vi "Station Wise.vi"(8 "error in (no error)":errorcluster, 11 "index":i32) -> (0 "error out":errorcluster, 2 "M":bool, 3 "S":bool)   [LabVIEW 2017]
uses:
  <vilib>/addons/database/Connection.llb/DB Tools Open Connec (Path).vi
  Globle/Current date.vi
  <vilib>/addons/database/NI_Database_API.lvlib
panel:
  in  "Cancel Button":bool
  out "G Ack 2":bool
  out "GL 2":bool
  out "Table 2":string[][](array[string])
  out "Table":string[][](array[string])
  out "Duration P":dbl format="%<%M:%S>t"
  out "Duration Q":dbl format="%<%M:%S>t"
  out "Duration M":dbl format="%<%M:%S>t"
  out "Duration L":dbl format="%<%M:%S>t"
  out "Duration GL":dbl format="%<%M:%S>t"
  out "COUNT P":i32
  out "COUNT  Q":i32
  out "COUNT  M":i32
  out "COUNT  Mat":i32
  out "P Ack":bool
  out "Q Ack":bool
  out "M Ack":bool
  out "L Ack":bool
  out "G Ack":bool
  out "SS":bool
  out "Q":bool
  out "M":bool
  out "COUNT Safety":i32
  out "P Duration Min":dbl format="%<%M:%S>t"
  out "Q Duration Min":dbl format="%<%M:%S>t"
  out "M Duration Min":dbl format="%<%M:%S>t"
  out "L Duration Min":dbl format="%<%M:%S>t"
  out "GL Duration min":dbl format="%<%M:%S>t"
  out "P Counter":i32
  out "Q Counter":i32
  out "M Counter":i32
  out "Mat Counter":i32
  out "Safety Counter":i32
  # "Station Wise Live Breakdown Status"
  # "Safety"
  # "Material"
  # "Maintenance"
  # "Quality"
  # "Startup/Setup"
  # "Stakeholder"
  # "Count"
  # "Duration"
  # "Station"
  # "Breakdown Name"
  # "Safety"
  # "Min"
  # "Breakdown"
  # "Material"
  # "Min"
  # "Acknowledgement"
  # "Maintenance"
  # "Min"
  # "Total Count"
  # "Quality"
  # "Min"
  # "Total Duration (Min)"
  # "Startup/Setup"
  # "Min"
  # "Designed And Developed By - Infinity Automation Systems Pvt. Ltd."
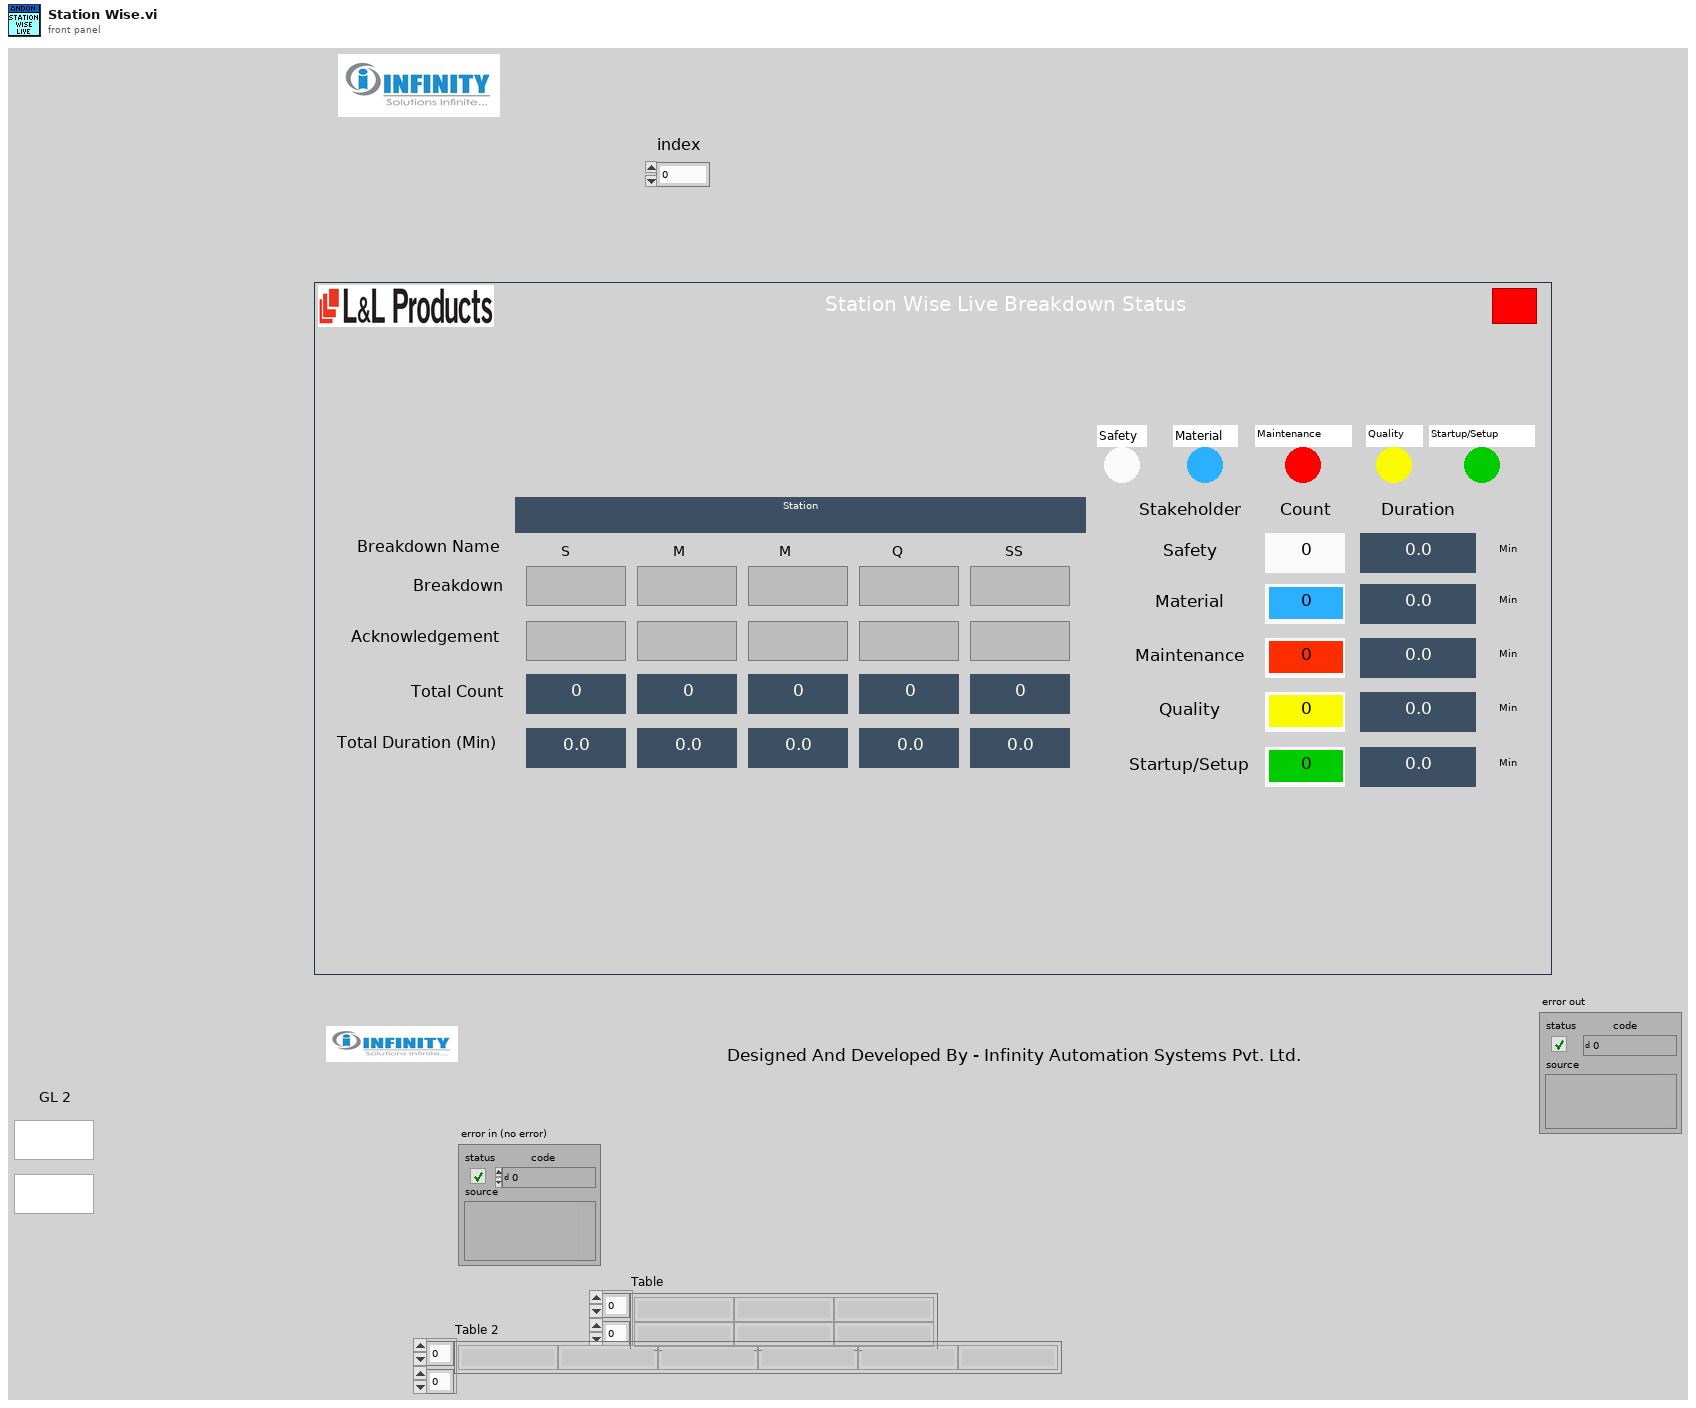
[diagram p1: front panel]
types:
  T1 = typedef "NI_Database_API.lvlib/Conn ObjectReference.ctl" = refnum<k1>
  T2 = enum32{"invalid app kind", "Development System", "Run Time System", "Student Edition", "Embedded LabVIEW", "Evaluation", "Custom"}
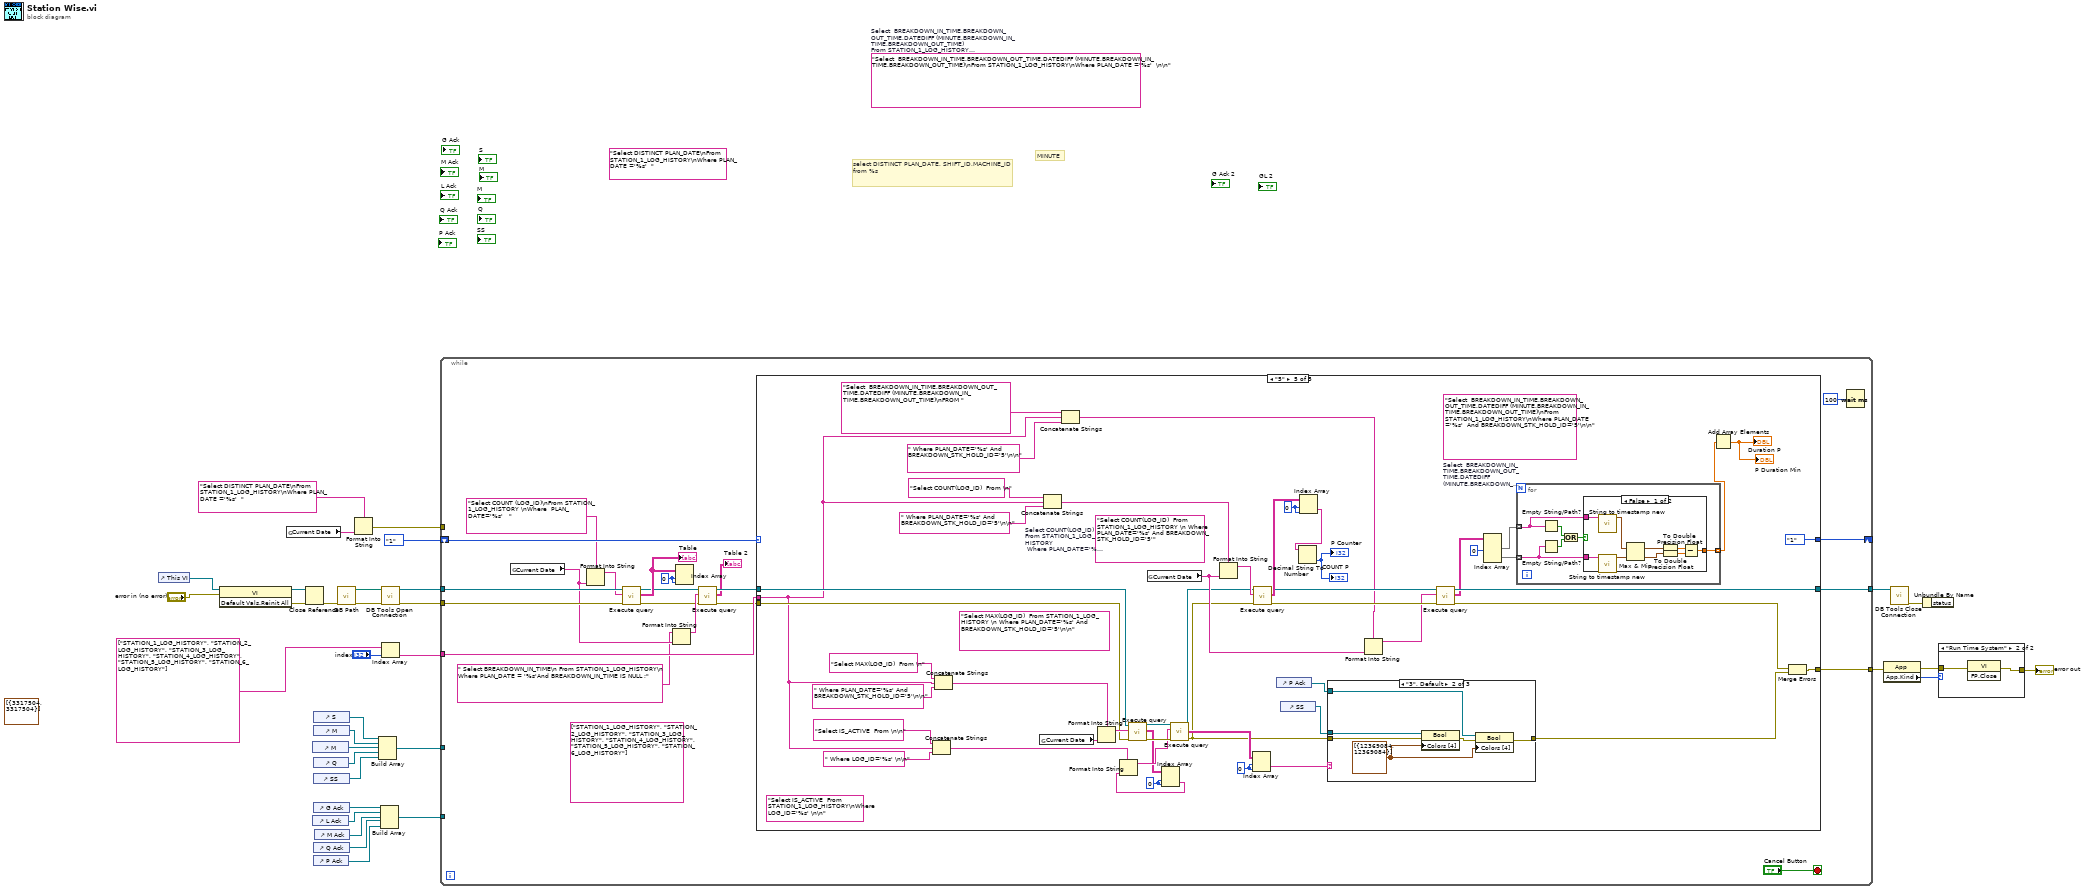
[diagram p0: block diagram]
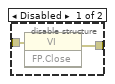
[diagram p3: hidden frame]
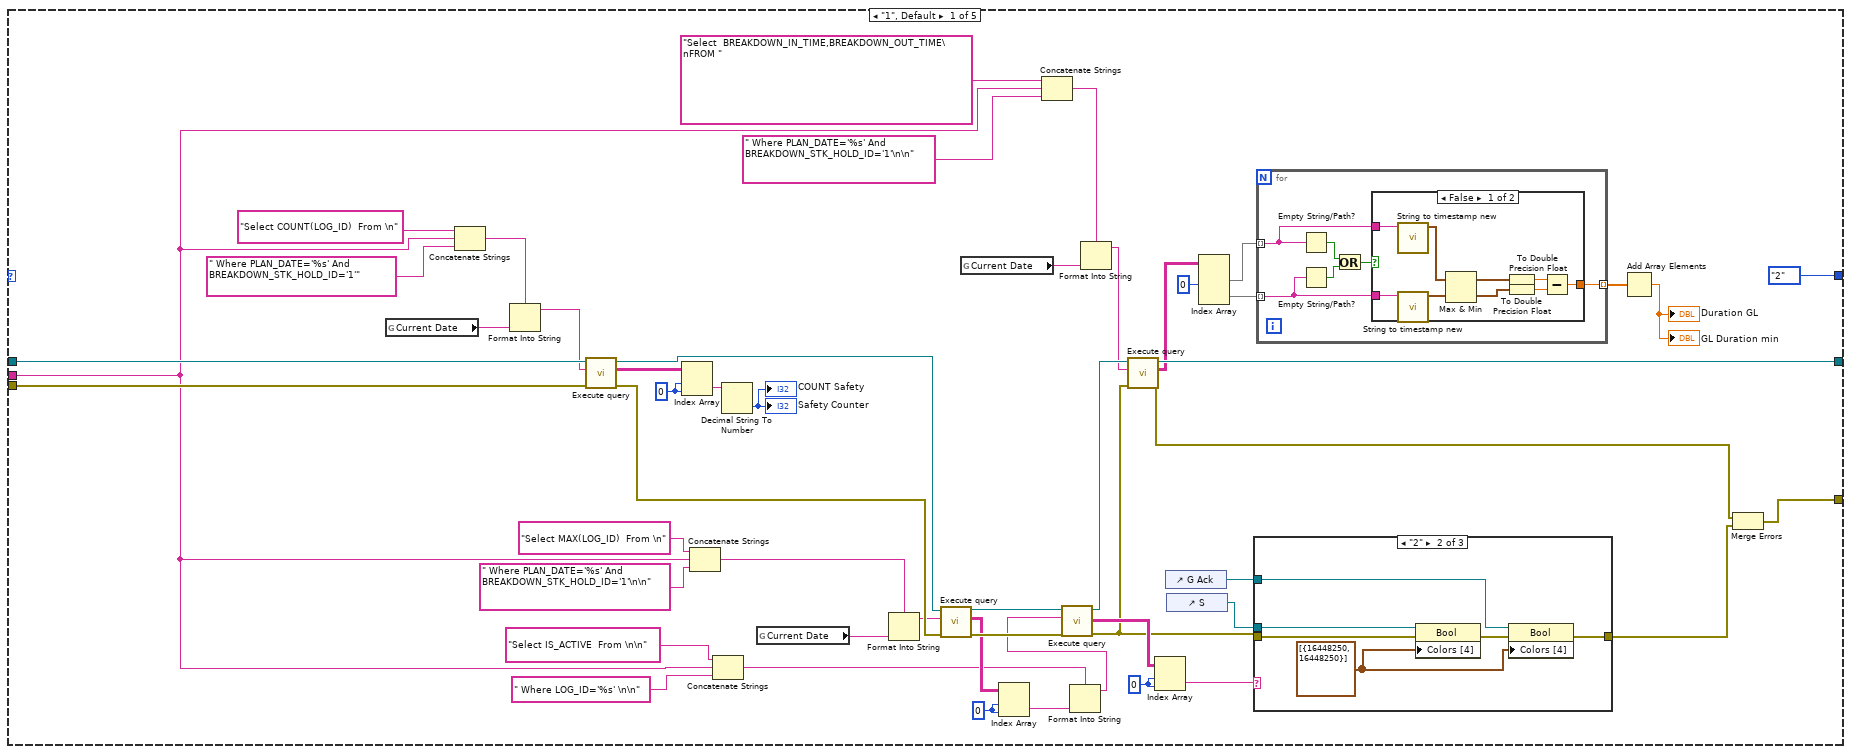
[diagram p4: hidden frame]
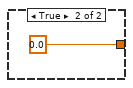
[diagram p5: hidden frame]
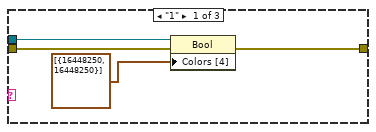
[diagram p6: hidden frame]
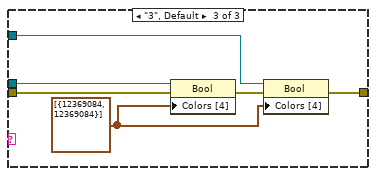
[diagram p7: hidden frame]
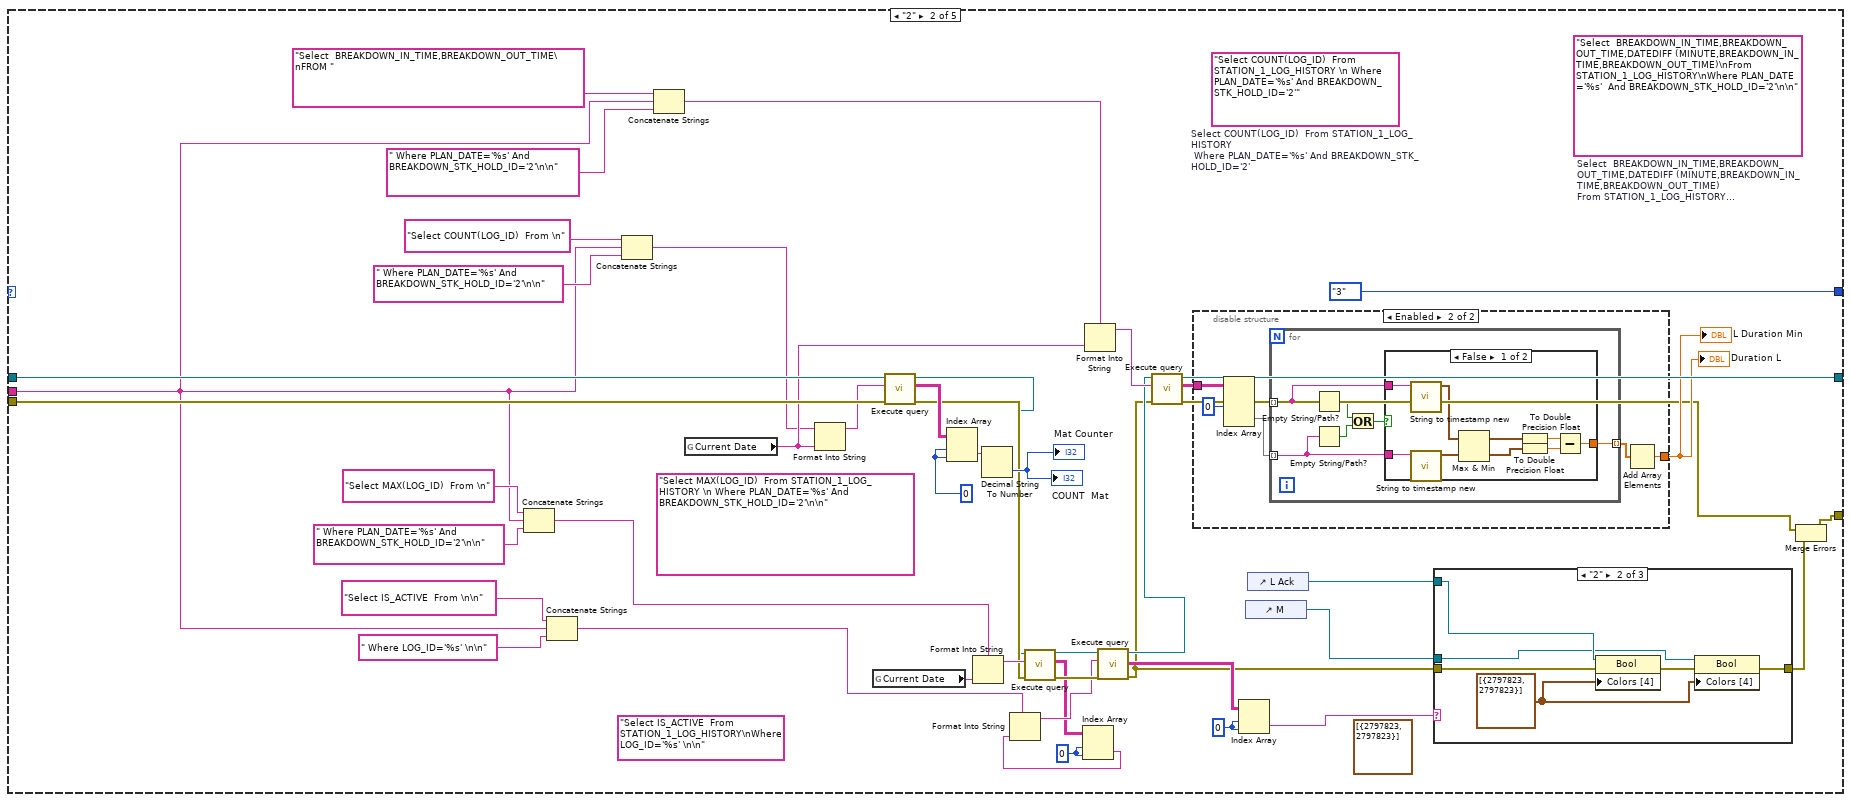
[diagram p8: hidden frame]
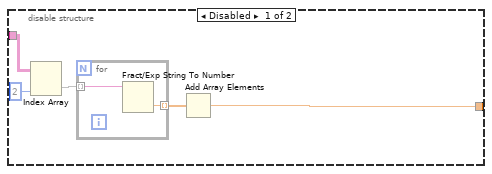
[diagram p9: hidden frame]
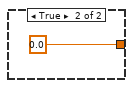
[diagram p10: hidden frame]
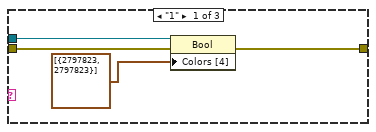
[diagram p11: hidden frame]
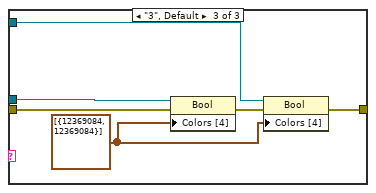
[diagram p12: hidden frame]
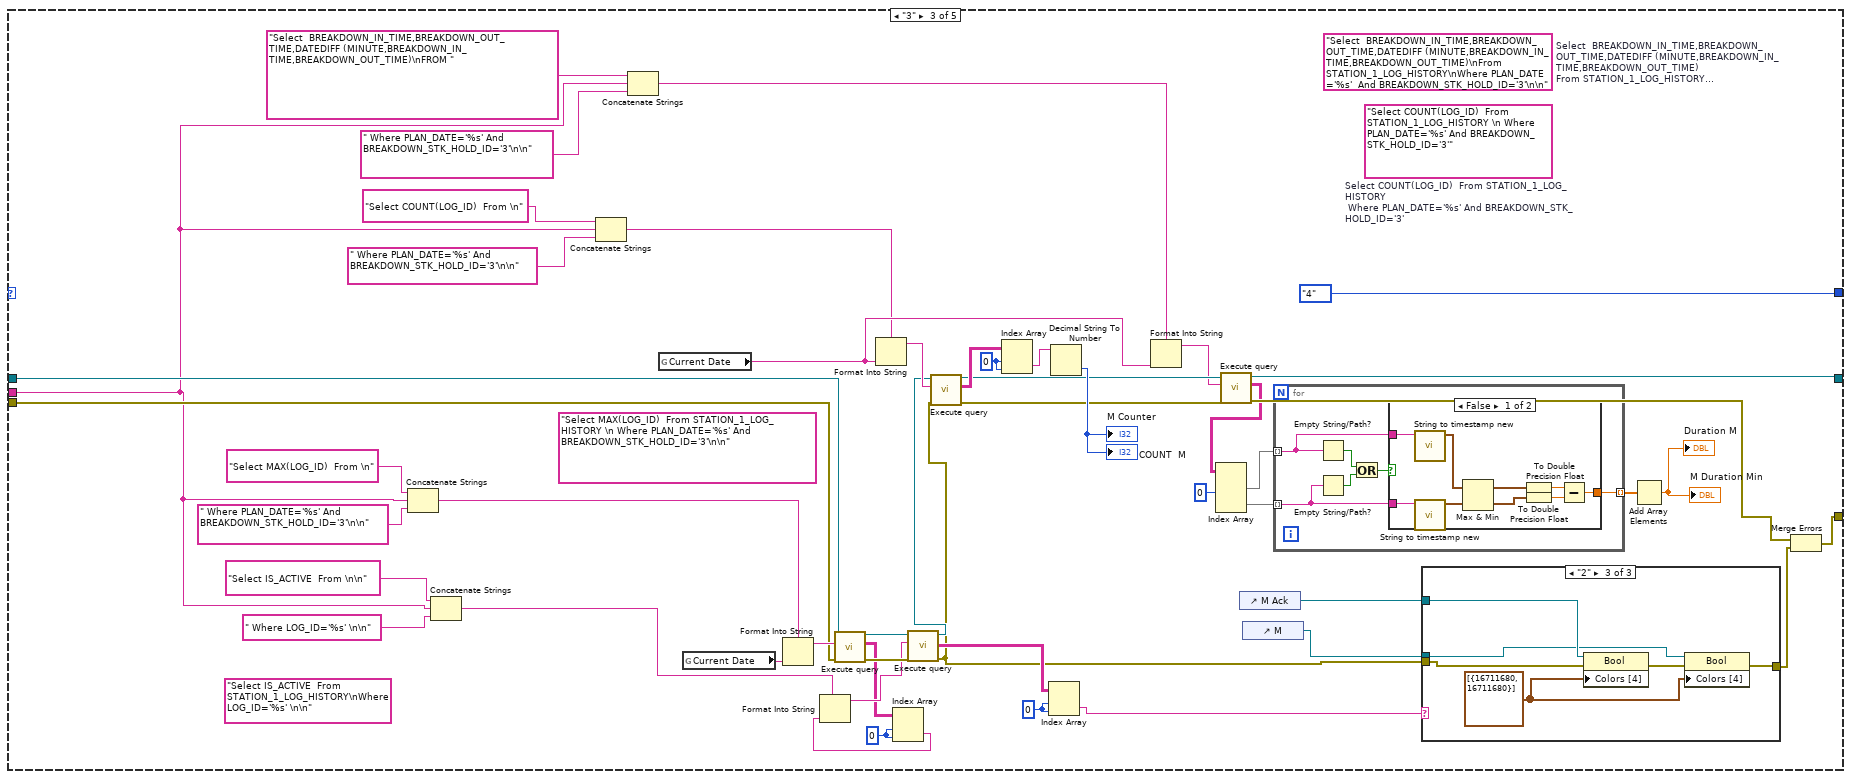
[diagram p13: hidden frame]
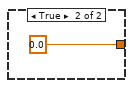
[diagram p14: hidden frame]
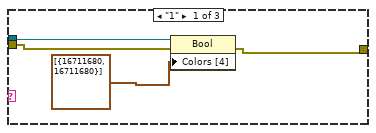
[diagram p15: hidden frame]
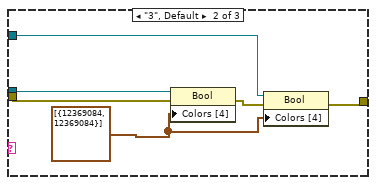
[diagram p16: hidden frame]
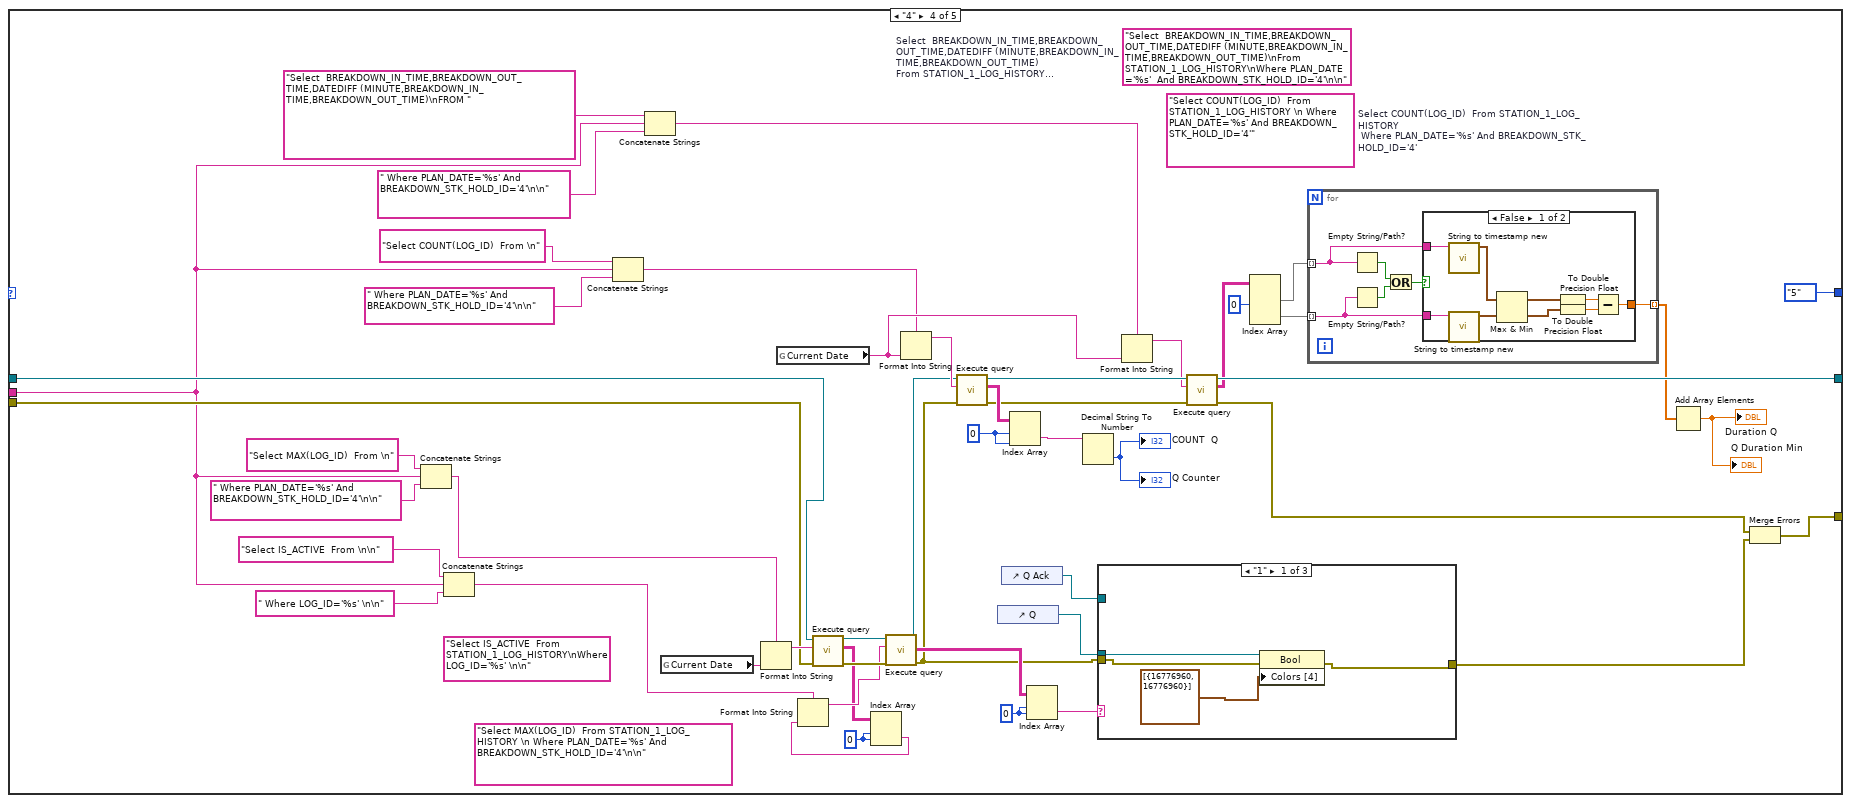
[diagram p17: hidden frame]
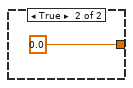
[diagram p18: hidden frame]
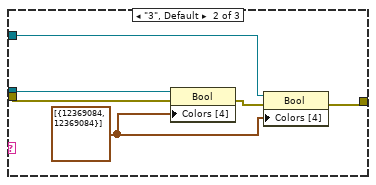
[diagram p19: hidden frame]
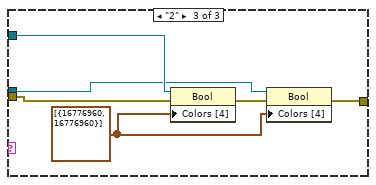
[diagram p20: hidden frame]
diagram:
  (unwired) "Select  BREAKDOWN_IN_TIME,BREAKDOWN_OUT_TIME,DATEDIFF (MINUTE,BREAKDOWN_IN_TIME,BREAKDOWN_OUT_TIME)\nFrom STATION_1_LOG_HISTORY\nWhere PLAN_DATE ='%s'  \n\n"  # Select  BREAKDOWN_IN_TIME,BREAKDOWN_OUT_TIME,DATEDIFF (MINUTE,BREAKDOWN_IN_TIME,BREAKDOWN_OUT_TIME) From STATION_1_LOG_HISTORY Where PLAN_DATE ='%s'
  (unwired) "Select DISTINCT PLAN_DATE\nFrom STATION_1_LOG_HISTORY\nWhere PLAN_DATE ='%s'  " ("format string")
  (unwired) cluster{u32, u32}[] [{3317504, 3317504}] ("Colors [4]")
  # "MINUTE"
  # "select DISTINCT PLAN_DATE, SHIFT_ID,MACHINE_ID\nfrom %s"
  n1 = control-ref of="This VI"() -> (w34:refnum<vi>)
  n2 = invoke class="VI" method="Default Vals.Reinit All"(reference=w34, error in="error in (no error)") -> (reference out=w32:refnum<vi>, error out=w33:errorcluster)  [unwired: 1 in, 1 out]
  n3 = global read "Current date.vi" "Current Date"() -> (w5:string)
  n4 = Close Reference(reference=w32, error in (no error)=w33) -> (error out=w28:errorcluster)
  n5 = control-ref of="M"() -> (w18:refnum<vi>)
  n6 = control-ref of="L Ack"() -> (w14:refnum<vi>)
  n7 = control-ref of="Q"() -> (w17:refnum<vi>)
  n8 = control-ref of="P Ack"() -> (w11:refnum<vi>)
  n9 = control-ref of="S"() -> (w20:refnum<vi>)
  n10 = control-ref of="M"() -> (w19:refnum<vi>)
  n11 = control-ref of="SS"() -> (w16:refnum<vi>)
  n12 = control-ref of="G Ack"() -> (w15:refnum<vi>)
  n13 = control-ref of="Q Ack"() -> (w12:refnum<vi>)
  n14 = control-ref of="M Ack"() -> (w13:refnum<vi>)
  n15 = call "DB Path.vi"("error in"=w28) -> ("error out"=w27:errorcluster, "DB Path"=w26:path)  [unwired: 9 in]
  n16 = Format Into String(format string="Select DISTINCT PLAN_DATE\nFrom STATION_1_LOG_HISTORY\nWhere PLAN_DATE ='%s'  ", w5) -> (error out=w3:errorcluster)  [unwired: 2 in, 1 out]
  n17 = Build Array(w20, w19, w18, w17, w16) -> (w10:refnum<vi>[])
  n18 = Build Array(w15, w14, w13, w12, w11) -> (w9:refnum<vi>[])
  n19 = call-poly <vilib>:"DB Tools Open Connection.vi"("error in (no error)"=w27, "connection information"=w26) -> ("error out"=w6:errorcluster, "connection reference"=w25:T1)  [unwired: 6 in]
  n20 = Index Array(array=string[] ["STATION_1_LOG_HISTORY", "STATION_2_LOG_HISTORY", "STATION_3_LOG_HISTORY", "STATION_4_LOG_HISTORY", "STATION_5_LOG_HISTORY", "STATION_6_LOG_HISTORY"], index="index") -> (element=w22:string)
  n21 = while {
    tunnel: w6 -> [w50]
    tunnel: [w55] -> w29
    tunnel: w25 -> [w51]
    tunnel: w22 -> [w48]
    shift-right: [w53] -> _
    shift-left: enum16{"1", "2", "3", "4", "5"}."1" -> [w54]
    tunnel: [w52] -> w2
    tunnel: w10 -> [_]
    tunnel: w9 -> [_]
    tunnel: w3 -> [_]
    stop <- "Cancel Button" stop-if-true
    (unwired) string[] ["STATION_1_LOG_HISTORY", "STATION_2_LOG_HISTORY", "STATION_3_LOG_HISTORY", "STATION_4_LOG_HISTORY", "STATION_5_LOG_HISTORY", "STATION_6_LOG_HISTORY"]
    w45 = 0 ("index (row)")
    n22 = global read "Current date.vi" "Current Date"() -> (w44:string)
    n23 = Format Into String(format string="Select COUNT (LOG_ID)\nFrom STATION_1_LOG_HISTORY \nWhere  PLAN_DATE='%s'   " ("string"), w44) -> (resulting string=w47:string)  [unwired: 2 in, 1 out]
    n24 = call "Execute query.vi"("error in (no error)"=w50, "String"=w47, "connection reference"=w51) -> ("error out"=w39:errorcluster, "Table"=w49:string[][], "connection reference 2"=w41:T1)  [unwired: 3 in, 3 out]
    "Table" <- w49
    n25 = Format Into String(format string=" Select BREAKDOWN_IN_TIME\n From STATION_1_LOG_HISTORY\n  Where PLAN_DATE = '%s'And BREAKDOWN_IN_TIME IS NULL ;" ("string"), w44) -> (resulting string=w42:string)  [unwired: 2 in, 1 out]
    n26 = Index Array(array=w49, index (row)=w45, index (col)=w45) -> ()  [unwired: 1 out]
    n27 = call "Execute query.vi"("error in (no error)"=w39, "String"=w42, "connection reference"=w41) -> ("error out"=w38:errorcluster, "Table"=→"Table 2":string[][], "connection reference 2"=w40:T1)  [unwired: 3 in, 3 out]
    n28 = case shown="\"5\"" w54 {
      tunnel: w38 -> [w100 w182 w254 w338 w421]
      tunnel: w40 -> [w106 w181 w253 w337 w420]
      tunnel: w48 -> [w68 w140 w236 w317 w402]
      tunnel: [w82 w155 w265 w330 w414] -> w55
      tunnel: [enum16{"1", "2", "3", "4", "5"}."2" enum16{"1", "2", "3", "4", "5"}."3" enum16{"1", "2", "3", "4", "5"}."4" enum16{"1", "2", "3", "4", "5"}."5" enum16{"1", "2", "3", "4", "5"}."1"] -> w53
      tunnel: [w101 w176 w271 w353 w435] -> w52
      frame "1", Default {
        w86 = 0 ("index (row)")
        w89 = 0 ("index (row)")
        w103 = 0 ("index (row)")
        n29 = global read "Current date.vi" "Current Date"() -> (w99:string)
        n30 = Concatenate Strings("Select COUNT(LOG_ID)  From \n", w68, " Where PLAN_DATE='%s' And BREAKDOWN_STK_HOLD_ID='1'") -> (w63:string)
        n31 = Format Into String(format string=w63, w99) -> (resulting string=w73:string)  [unwired: 2 in, 1 out]
        n32 = call "Execute query.vi"("error in (no error)"=w100, "String"=w73, "connection reference"=w106) -> ("error out"=w96:errorcluster, "Table"=w98:string[][], "connection reference 2"=w94:T1)  [unwired: 3 in, 3 out]
        n33 = Index Array(array=w98, index (row)=w103, index (col)=w103) -> (element=w102:string)
        n34 = Concatenate Strings("Select MAX(LOG_ID)  From \n", w68, " Where PLAN_DATE='%s' And BREAKDOWN_STK_HOLD_ID='1'\n\n") -> (w62:string)
        n35 = Concatenate Strings("Select IS_ACTIVE  From \n\n", w68, " Where LOG_ID='%s' \n\n") -> (w65:string)
        n36 = Decimal String To Number(string=w102) -> (number=→"Safety Counter" →"COUNT Safety":i32)  [unwired: 2 in, 1 out]
        n37 = global read "Current date.vi" "Current Date"() -> (w97:string)
        n38 = Format Into String(format string=w62, w97) -> (resulting string=w95:string)  [unwired: 2 in, 1 out]
        n39 = call "Execute query.vi"("error in (no error)"=w96, "String"=w95, "connection reference"=w94) -> ("error out"=w93:errorcluster, "Table"=w88:string[][], "connection reference 2"=w92:T1)  [unwired: 3 in, 3 out]
        n40 = global read "Current date.vi" "Current Date"() -> (w75:string)
        n41 = Index Array(array=w88, index (row)=w89, index (col)=w89) -> (element=w87:string)
        n42 = Concatenate Strings("Select  BREAKDOWN_IN_TIME,BREAKDOWN_OUT_TIME\nFROM " ("SQL query"), w68, " Where PLAN_DATE='%s' And BREAKDOWN_STK_HOLD_ID='1'\n\n") -> (w64:string)
        n43 = Format Into String(format string=w65, w87) -> (resulting string=w90:string)  [unwired: 2 in, 1 out]
        n44 = call "Execute query.vi"("error in (no error)"=w93, "String"=w90, "connection reference"=w92) -> ("error out"=w84:errorcluster, "Table"=w85:string[][], "connection reference 2"=w91:T1)  [unwired: 3 in, 3 out]
        n45 = Format Into String(format string=w64, w75) -> (resulting string=w74:string)  [unwired: 2 in, 1 out]
        n46 = call "Execute query.vi"("error in (no error)"=w84, "String"=w74, "connection reference"=w91) -> ("error out"=w83:errorcluster, "Table"=w61:string[][], "connection reference 2"=w101:T1)  [unwired: 3 in, 3 out]
        n47 = Index Array(array=w85, index (row)=w86, index (col)=w86) -> (element=w78:string)
        n48 = control-ref of="G Ack"() -> (w79:refnum<vi>)
        n49 = control-ref of="S"() -> (w80:refnum<vi>)
        n50 = Index Array(array=w61, index (col) #1=0 ("disabled index (col)")) -> (element #1=w59:string[], element #2=w58:string[])  [unwired: 3 in]
        n51 = case shown="\"2\"" w78 {
          tunnel: w84 -> [w126 w132 w138]
          tunnel: [w124 w129 w135] -> w81
          tunnel: w80 -> [w123 w128 w134]
          tunnel: w79 -> [_ w127 w133]
          frame "1" {
            n52 = property class="Bool"(reference=w123, error in=w126, "Colors [4]"=cluster{u32, u32}[] [{16448250, 16448250}]) -> (error out=w124:errorcluster)  [unwired: 1 out]
          }
          frame "2" {
            w130 = cluster{u32, u32}[] [{16448250, 16448250}] ("Colors [4]")
            n53 = property class="Bool"(reference=w128, error in=w132, "Colors [4]"=w130) -> (error out=w131:errorcluster)  [unwired: 1 out]
            n54 = property class="Bool"(reference=w127, error in=w131, "Colors [4]"=w130) -> (error out=w129:errorcluster)  [unwired: 1 out]
          }
          frame "3", Default {
            w136 = cluster{u32, u32}[] [{12369084, 12369084}] ("Colors [4]")
            n55 = property class="Bool"(reference=w134, error in=w138, "Colors [4]"=w136) -> (error out=w137:errorcluster)  [unwired: 1 out]
            n56 = property class="Bool"(reference=w133, error in=w137, "Colors [4]"=w136) -> (error out=w135:errorcluster)  [unwired: 1 out]
          }
        }
        n57 = for {
          tunnel: w59 -> [w108] mode=indexing
          tunnel: w58 -> [w109] mode=indexing
          tunnel: [w107] -> w57 mode=indexing
          n58 = Empty String/Path?(string/path=w108) -> (empty?=w111:bool)
          n59 = Empty String/Path?(string/path=w109) -> (empty?=w112:bool)
          n60 = Or(x=w111, y=w112) -> (x .or. y?=w110:bool)
          n61 = case shown="False" w110 {
            tunnel: [w115 0.0] -> w107
            tunnel: w108 -> [w114 _]
            tunnel: w109 -> [w113 _]
            frame False {
              n62 = call "String to timestamp new.vi"("String Timestamp"=w114) -> ("Timestamp"=w117:timestamp)  [unwired: 10 in]
              n63 = call "String to timestamp new.vi"("String Timestamp"=w113) -> ("Timestamp"=w116:timestamp)  [unwired: 10 in]
              n64 = Max & Min(x=w117, y=w116) -> (max(x,y)=w121:timestamp, min(x,y)=w120:timestamp)
              n65 = To Double Precision Float(number=w121) -> (double precision float=w119:dbl)
              n66 = To Double Precision Float(number=w120) -> (double precision float=w118:dbl)
              n67 = Subtract(x=w119, y=w118) -> (x-y=w115:dbl)
            }
            frame True {
            }
          }
        }
        n68 = Add Array Elements(numeric array=w57) -> (sum=→"GL Duration min" →"Duration GL":dbl)
        n69 = Merge Errors(w83, w81) -> (w82:errorcluster)
      }
      frame "2" {
        (unwired) cluster{u32, u32}[] [{2797823, 2797823}] ("Colors [4]")
        w164 = 0 ("index (row)")
        w167 = 0 ("index (row)")
        (unwired) "Select IS_ACTIVE  From STATION_1_LOG_HISTORY\nWhere LOG_ID='%s' \n\n"
        (unwired) "Select MAX(LOG_ID)  From STATION_1_LOG_HISTORY \n Where PLAN_DATE='%s' And BREAKDOWN_STK_HOLD_ID='2'\n\n"
        (unwired) "Select  BREAKDOWN_IN_TIME,BREAKDOWN_OUT_TIME,DATEDIFF (MINUTE,BREAKDOWN_IN_TIME,BREAKDOWN_OUT_TIME)\nFrom STATION_1_LOG_HISTORY\nWhere PLAN_DATE ='%s'  And BREAKDOWN_STK_HOLD_ID='2'\n\n"  # Select  BREAKDOWN_IN_TIME,BREAKDOWN_OUT_TIME,DATEDIFF (MINUTE,BREAKDOWN_IN_TIME,BREAKDOWN_OUT_TIME) From STATION_1_LOG_HISTORY Where PLAN_DATE ='%s'  And BREAKDOWN_STK_HOLD_ID='2'
        w178 = 0 ("index (row)")
        (unwired) "Select COUNT(LOG_ID)  From STATION_1_LOG_HISTORY \n Where PLAN_DATE='%s' And BREAKDOWN_STK_HOLD_ID='2'"  # Select COUNT(LOG_ID)  From STATION_1_LOG_HISTORY   Where PLAN_DATE='%s' And BREAKDOWN_STK_HOLD_ID='2'
        n70 = Concatenate Strings("Select MAX(LOG_ID)  From \n", w140, " Where PLAN_DATE='%s' And BREAKDOWN_STK_HOLD_ID='2'\n\n") -> (w142:string)
        n71 = Concatenate Strings("Select IS_ACTIVE  From \n\n", w140, " Where LOG_ID='%s' \n\n") -> (w141:string)
        n72 = Concatenate Strings("Select COUNT(LOG_ID)  From \n", w140, " Where PLAN_DATE='%s' And BREAKDOWN_STK_HOLD_ID='2'\n\n") -> (w147:string)
        n73 = Concatenate Strings("Select  BREAKDOWN_IN_TIME,BREAKDOWN_OUT_TIME\nFROM " ("SQL query"), w140, " Where PLAN_DATE='%s' And BREAKDOWN_STK_HOLD_ID='2'\n\n") -> (w150:string)
        n74 = global read "Current date.vi" "Current Date"() -> (w175:string)
        n75 = Format Into String(format string=w147, w175) -> (resulting string=w180:string)  [unwired: 2 in, 1 out]
        n76 = global read "Current date.vi" "Current Date"() -> (w172:string)
        n77 = call "Execute query.vi"("error in (no error)"=w182, "String"=w180, "connection reference"=w181) -> ("error out"=w162:errorcluster, "Table"=w179:string[][], "connection reference 2"=w160:T1)  [unwired: 3 in, 3 out]
        n78 = Index Array(array=w179, index (row)=w178, index (col)=w178) -> (element=w177:string)
        n79 = Format Into String(format string=w142, w172) -> (resulting string=w171:string)  [unwired: 2 in, 1 out]
        n80 = Decimal String To Number(string=w177) -> (number=→"Mat Counter" →"COUNT  Mat":i32)  [unwired: 2 in, 1 out]
        n81 = call "Execute query.vi"("error in (no error)"=w162, "String"=w171, "connection reference"=w160) -> ("error out"=w170:errorcluster, "Table"=w166:string[][], "connection reference 2"=w169:T1)  [unwired: 3 in, 3 out]
        n82 = Index Array(array=w166, index (row)=w167, index (col)=w167) -> (element=w165:string)
        n83 = Format Into String(format string=w141, w165) -> (resulting string=w168:string)  [unwired: 2 in, 1 out]
        n84 = Format Into String(format string=w150, w175) -> (resulting string=w174:string)  [unwired: 2 in, 1 out]
        n85 = call "Execute query.vi"("error in (no error)"=w170, "String"=w168, "connection reference"=w169) -> ("error out"=w158:errorcluster, "Table"=w163:string[][], "connection reference 2"=w161:T1)  [unwired: 3 in, 3 out]
        n86 = call "Execute query.vi"("error in (no error)"=w158, "String"=w174, "connection reference"=w161) -> ("error out"=w156:errorcluster, "Table"=w139:string[][], "connection reference 2"=w176:T1)  [unwired: 3 in, 3 out]
        n87 = disable-structure shown="Enabled" {
          disable-tunnel: [w186 w193] -> w173
          disable-tunnel: w139 -> [w185 w197]
          frame Disabled {
            n88 = Index Array(array=w185, index (col)=2 ("disabled index (col)")) -> (element=w187:string[])  [unwired: 1 in]
            n89 = for {
              tunnel: w187 -> [w191] mode=indexing
              tunnel: [w190] -> w189 mode=indexing
              n90 = Fract/Exp String To Number(string=w191) -> (number=w190:dbl)  [unwired: 3 in, 1 out]
            }
            n91 = Add Array Elements(numeric array=w189) -> (sum=w186:dbl)
          }
          frame Enabled {
            n92 = Index Array(array=w197, index (col) #1=0 ("disabled index (col)")) -> (element #1=w195:string[], element #2=w194:string[])  [unwired: 3 in]
            n93 = for {
              tunnel: w195 -> [w199] mode=indexing
              tunnel: w194 -> [w200] mode=indexing
              tunnel: [w198] -> w192 mode=indexing
              n94 = Empty String/Path?(string/path=w199) -> (empty?=w202:bool)
              n95 = Empty String/Path?(string/path=w200) -> (empty?=w203:bool)
              n96 = Or(x=w202, y=w203) -> (x .or. y?=w201:bool)
              n97 = case shown="False" w201 {
                tunnel: [w206 0.0] -> w198
                tunnel: w199 -> [w205 _]
                tunnel: w200 -> [w204 _]
                frame False {
                  n98 = call "String to timestamp new.vi"("String Timestamp"=w205) -> ("Timestamp"=w208:timestamp)  [unwired: 10 in]
                  n99 = call "String to timestamp new.vi"("String Timestamp"=w204) -> ("Timestamp"=w207:timestamp)  [unwired: 10 in]
                  n100 = Max & Min(x=w208, y=w207) -> (max(x,y)=w212:timestamp, min(x,y)=w211:timestamp)
                  n101 = To Double Precision Float(number=w212) -> (double precision float=w210:dbl)
                  n102 = To Double Precision Float(number=w211) -> (double precision float=w209:dbl)
                  n103 = Subtract(x=w210, y=w209) -> (x-y=w206:dbl)
                }
                frame True {
                }
              }
            }
            n104 = Add Array Elements(numeric array=w192) -> (sum=w193:dbl)
          }
        }
        "L Duration Min" <- w173
        "Duration L" <- w173
        n105 = Index Array(array=w163, index (row)=w164, index (col)=w164) -> (element=w159:string)
        n106 = control-ref of="M"() -> (w154:refnum<vi>)
        n107 = control-ref of="L Ack"() -> (w153:refnum<vi>)
        n108 = case shown="\"2\"" w159 {
          tunnel: w158 -> [w217 w223 w229]
          tunnel: [w214 w219 w226] -> w157
          tunnel: w154 -> [w215 w221 w225]
          tunnel: w153 -> [_ w222 w224]
          frame "1" {
            n109 = property class="Bool"(reference=w215, error in=w217, "Colors [4]"=cluster{u32, u32}[] [{2797823, 2797823}]) -> (error out=w214:errorcluster)  [unwired: 1 out]
          }
          frame "2" {
            w218 = cluster{u32, u32}[] [{2797823, 2797823}] ("Colors [4]")
            n110 = property class="Bool"(reference=w222, error in=w223, "Colors [4]"=w218) -> (error out=w220:errorcluster)  [unwired: 1 out]
            n111 = property class="Bool"(reference=w221, error in=w220, "Colors [4]"=w218) -> (error out=w219:errorcluster)  [unwired: 1 out]
          }
          frame "3", Default {
            w227 = cluster{u32, u32}[] [{12369084, 12369084}] ("Colors [4]")
            n112 = property class="Bool"(reference=w225, error in=w229, "Colors [4]"=w227) -> (error out=w228:errorcluster)  [unwired: 1 out]
            n113 = property class="Bool"(reference=w224, error in=w228, "Colors [4]"=w227) -> (error out=w226:errorcluster)  [unwired: 1 out]
          }
        }
        n114 = Merge Errors(w156, w157) -> (w155:errorcluster)
      }
      frame "3" {
        w256 = 0 ("index (row)")
        w259 = 0 ("index (row)")
        (unwired) "Select IS_ACTIVE  From STATION_1_LOG_HISTORY\nWhere LOG_ID='%s' \n\n"
        (unwired) "Select MAX(LOG_ID)  From STATION_1_LOG_HISTORY \n Where PLAN_DATE='%s' And BREAKDOWN_STK_HOLD_ID='3'\n\n"
        (unwired) "Select  BREAKDOWN_IN_TIME,BREAKDOWN_OUT_TIME,DATEDIFF (MINUTE,BREAKDOWN_IN_TIME,BREAKDOWN_OUT_TIME)\nFrom STATION_1_LOG_HISTORY\nWhere PLAN_DATE ='%s'  And BREAKDOWN_STK_HOLD_ID='3'\n\n"  # Select  BREAKDOWN_IN_TIME,BREAKDOWN_OUT_TIME,DATEDIFF (MINUTE,BREAKDOWN_IN_TIME,BREAKDOWN_OUT_TIME) From STATION_1_LOG_HISTORY Where PLAN_DATE ='%s'  And BREAKDOWN_STK_HOLD_ID='3'
        w275 = 0 ("index (row)")
        (unwired) "Select COUNT(LOG_ID)  From STATION_1_LOG_HISTORY \n Where PLAN_DATE='%s' And BREAKDOWN_STK_HOLD_ID='3'"  # Select COUNT(LOG_ID)  From STATION_1_LOG_HISTORY   Where PLAN_DATE='%s' And BREAKDOWN_STK_HOLD_ID='3'
        n115 = Concatenate Strings("Select MAX(LOG_ID)  From \n", w236, " Where PLAN_DATE='%s' And BREAKDOWN_STK_HOLD_ID='3'\n\n") -> (w237:string)
        n116 = Concatenate Strings("Select IS_ACTIVE  From \n\n", w236, " Where LOG_ID='%s' \n\n") -> (w235:string)
        n117 = Concatenate Strings("Select COUNT(LOG_ID)  From \n", w236, " Where PLAN_DATE='%s' And BREAKDOWN_STK_HOLD_ID='3'\n\n") -> (w242:string)
        n118 = Concatenate Strings("Select  BREAKDOWN_IN_TIME,BREAKDOWN_OUT_TIME,DATEDIFF (MINUTE,BREAKDOWN_IN_TIME,BREAKDOWN_OUT_TIME)\nFROM " ("SQL query"), w236, " Where PLAN_DATE='%s' And BREAKDOWN_STK_HOLD_ID='3'\n\n") -> (w243:string)
        n119 = global read "Current date.vi" "Current Date"() -> (w270:string)
        n120 = global read "Current date.vi" "Current Date"() -> (w264:string)
        n121 = Format Into String(format string=w237, w264) -> (resulting string=w263:string)  [unwired: 2 in, 1 out]
        n122 = call "Execute query.vi"("error in (no error)"=w254, "String"=w263, "connection reference"=w253) -> ("error out"=w262:errorcluster, "Table"=w258:string[][], "connection reference 2"=w261:T1)  [unwired: 3 in, 3 out]
        n123 = Format Into String(format string=w242, w270) -> (resulting string=w277:string)  [unwired: 2 in, 1 out]
        n124 = Index Array(array=w258, index (row)=w259, index (col)=w259) -> (element=w257:string)
        n125 = Format Into String(format string=w235, w257) -> (resulting string=w260:string)  [unwired: 2 in, 1 out]
        n126 = call "Execute query.vi"("error in (no error)"=w262, "String"=w260, "connection reference"=w261) -> ("error out"=w248:errorcluster, "Table"=w255:string[][], "connection reference 2"=w252:T1)  [unwired: 3 in, 3 out]
        n127 = call "Execute query.vi"("error in (no error)"=w248, "String"=w277, "connection reference"=w252) -> ("error out"=w273:errorcluster, "Table"=w276:string[][], "connection reference 2"=w272:T1)  [unwired: 3 in, 3 out]
        n128 = Index Array(array=w276, index (row)=w275, index (col)=w275) -> (element=w274:string)
        n129 = Index Array(array=w255, index (row)=w256, index (col)=w256) -> (element=w251:string)
        n130 = Decimal String To Number(string=w274) -> (number=→"M Counter" →"COUNT  M":i32)  [unwired: 2 in, 1 out]
        n131 = Format Into String(format string=w243, w270) -> (resulting string=w269:string)  [unwired: 2 in, 1 out]
        n132 = call "Execute query.vi"("error in (no error)"=w273, "String"=w269, "connection reference"=w272) -> ("error out"=w266:errorcluster, "Table"=w230:string[][], "connection reference 2"=w271:T1)  [unwired: 3 in, 3 out]
        n133 = Index Array(array=w230, index (col) #1=0 ("disabled index (col)")) -> (element #1=w233:string[], element #2=w232:string[])  [unwired: 3 in]
        n134 = control-ref of="M Ack"() -> (w250:refnum<vi>)
        n135 = control-ref of="M"() -> (w249:refnum<vi>)
        n136 = for {
          tunnel: w233 -> [w281] mode=indexing
          tunnel: w232 -> [w282] mode=indexing
          tunnel: [w280] -> w231 mode=indexing
          n137 = Empty String/Path?(string/path=w281) -> (empty?=w284:bool)
          n138 = Empty String/Path?(string/path=w282) -> (empty?=w285:bool)
          n139 = Or(x=w284, y=w285) -> (x .or. y?=w283:bool)
          n140 = case shown="False" w283 {
            tunnel: [w288 0.0] -> w280
            tunnel: w281 -> [w287 _]
            tunnel: w282 -> [w286 _]
            frame False {
              n141 = call "String to timestamp new.vi"("String Timestamp"=w287) -> ("Timestamp"=w290:timestamp)  [unwired: 10 in]
              n142 = call "String to timestamp new.vi"("String Timestamp"=w286) -> ("Timestamp"=w289:timestamp)  [unwired: 10 in]
              n143 = Max & Min(x=w290, y=w289) -> (max(x,y)=w294:timestamp, min(x,y)=w293:timestamp)
              n144 = To Double Precision Float(number=w294) -> (double precision float=w292:dbl)
              n145 = To Double Precision Float(number=w293) -> (double precision float=w291:dbl)
              n146 = Subtract(x=w292, y=w291) -> (x-y=w288:dbl)
            }
            frame True {
            }
          }
        }
        n147 = case shown="\"2\"" w251 {
          tunnel: [w296 w303 w308] -> w267
          tunnel: w250 -> [_ w302 w310]
          tunnel: w249 -> [w297 w301 w307]
          tunnel: w248 -> [w298 w300 w311]
          frame "1" {
            n148 = property class="Bool"(reference=w297, error in=w298, "Colors [4]"=cluster{u32, u32}[] [{16711680, 16711680}]) -> (error out=w296:errorcluster)  [unwired: 1 out]
          }
          frame "3", Default {
            w304 = cluster{u32, u32}[] [{12369084, 12369084}] ("Colors [4]")
            n149 = property class="Bool"(reference=w301, error in=w300, "Colors [4]"=w304) -> (error out=w305:errorcluster)  [unwired: 1 out]
            n150 = property class="Bool"(reference=w302, error in=w305, "Colors [4]"=w304) -> (error out=w303:errorcluster)  [unwired: 1 out]
          }
          frame "2" {
            w306 = cluster{u32, u32}[] [{16711680, 16711680}] ("Colors [4]")
            n151 = property class="Bool"(reference=w310, error in=w311, "Colors [4]"=w306) -> (error out=w309:errorcluster)  [unwired: 1 out]
            n152 = property class="Bool"(reference=w307, error in=w309, "Colors [4]"=w306) -> (error out=w308:errorcluster)  [unwired: 1 out]
          }
        }
        n153 = Add Array Elements(numeric array=w231) -> (sum=→"M Duration Min" →"Duration M":dbl)
        n154 = Merge Errors(w266, w267) -> (w265:errorcluster)
      }
      frame "4" {
        w340 = 0 ("index (row)")
        w339 = 0 ("index (row)")
        (unwired) "Select IS_ACTIVE  From STATION_1_LOG_HISTORY\nWhere LOG_ID='%s' \n\n"
        (unwired) "Select MAX(LOG_ID)  From STATION_1_LOG_HISTORY \n Where PLAN_DATE='%s' And BREAKDOWN_STK_HOLD_ID='4'\n\n"
        (unwired) "Select  BREAKDOWN_IN_TIME,BREAKDOWN_OUT_TIME,DATEDIFF (MINUTE,BREAKDOWN_IN_TIME,BREAKDOWN_OUT_TIME)\nFrom STATION_1_LOG_HISTORY\nWhere PLAN_DATE ='%s'  And BREAKDOWN_STK_HOLD_ID='4'\n\n"  # Select  BREAKDOWN_IN_TIME,BREAKDOWN_OUT_TIME,DATEDIFF (MINUTE,BREAKDOWN_IN_TIME,BREAKDOWN_OUT_TIME) From STATION_1_LOG_HISTORY Where PLAN_DATE ='%s'  And BREAKDOWN_STK_HOLD_ID='4'
        w357 = 0 ("index (row)")
        (unwired) "Select COUNT(LOG_ID)  From STATION_1_LOG_HISTORY \n Where PLAN_DATE='%s' And BREAKDOWN_STK_HOLD_ID='4'"  # Select COUNT(LOG_ID)  From STATION_1_LOG_HISTORY   Where PLAN_DATE='%s' And BREAKDOWN_STK_HOLD_ID='4'
        n155 = Concatenate Strings("Select MAX(LOG_ID)  From \n", w317, " Where PLAN_DATE='%s' And BREAKDOWN_STK_HOLD_ID='4'\n\n") -> (w319:string)
        n156 = Concatenate Strings("Select IS_ACTIVE  From \n\n", w317, " Where LOG_ID='%s' \n\n") -> (w318:string)
        n157 = Concatenate Strings("Select COUNT(LOG_ID)  From \n", w317, " Where PLAN_DATE='%s' And BREAKDOWN_STK_HOLD_ID='4'\n\n") -> (w324:string)
        n158 = Concatenate Strings("Select  BREAKDOWN_IN_TIME,BREAKDOWN_OUT_TIME,DATEDIFF (MINUTE,BREAKDOWN_IN_TIME,BREAKDOWN_OUT_TIME)\nFROM " ("SQL query"), w317, " Where PLAN_DATE='%s' And BREAKDOWN_STK_HOLD_ID='4'\n\n") -> (w325:string)
        n159 = global read "Current date.vi" "Current Date"() -> (w348:string)
        n160 = Format Into String(format string=w319, w348) -> (resulting string=w347:string)  [unwired: 2 in, 1 out]
        n161 = global read "Current date.vi" "Current Date"() -> (w352:string)
        n162 = call "Execute query.vi"("error in (no error)"=w338, "String"=w347, "connection reference"=w337) -> ("error out"=w346:errorcluster, "Table"=w343:string[][], "connection reference 2"=w345:T1)  [unwired: 3 in, 3 out]
        n163 = Index Array(array=w343, index (row)=w339, index (col)=w339) -> (element=w342:string)
        n164 = Format Into String(format string=w318, w342) -> (resulting string=w344:string)  [unwired: 2 in, 1 out]
        n165 = call "Execute query.vi"("error in (no error)"=w346, "String"=w344, "connection reference"=w345) -> ("error out"=w335:errorcluster, "Table"=w341:string[][], "connection reference 2"=w336:T1)  [unwired: 3 in, 3 out]
        n166 = Format Into String(format string=w324, w352) -> (resulting string=w359:string)  [unwired: 2 in, 1 out]
        n167 = call "Execute query.vi"("error in (no error)"=w335, "String"=w359, "connection reference"=w336) -> ("error out"=w355:errorcluster, "Table"=w358:string[][], "connection reference 2"=w354:T1)  [unwired: 3 in, 3 out]
        n168 = control-ref of="Q"() -> (w334:refnum<vi>)
        n169 = control-ref of="Q Ack"() -> (w333:refnum<vi>)
        n170 = Index Array(array=w358, index (row)=w357, index (col)=w357) -> (element=w356:string)
        n171 = Index Array(array=w341, index (row)=w340, index (col)=w340) -> (element=w349:string)
        n172 = Decimal String To Number(string=w356) -> (number=→"Q Counter" →"COUNT  Q":i32)  [unwired: 2 in, 1 out]
        n173 = case shown="\"1\"" w349 {
          tunnel: [w378 w385 w391] -> w331
          tunnel: w333 -> [_ w384 w392]
          tunnel: w334 -> [w379 w383 w389]
          tunnel: w335 -> [w380 w382 w393]
          frame "1" {
            n174 = property class="Bool"(reference=w379, error in=w380, "Colors [4]"=cluster{u32, u32}[] [{16776960, 16776960}]) -> (error out=w378:errorcluster)  [unwired: 1 out]
          }
          frame "3", Default {
            w386 = cluster{u32, u32}[] [{12369084, 12369084}] ("Colors [4]")
            n175 = property class="Bool"(reference=w383, error in=w382, "Colors [4]"=w386) -> (error out=w387:errorcluster)  [unwired: 1 out]
            n176 = property class="Bool"(reference=w384, error in=w387, "Colors [4]"=w386) -> (error out=w385:errorcluster)  [unwired: 1 out]
          }
          frame "2" {
            w388 = cluster{u32, u32}[] [{16776960, 16776960}] ("Colors [4]")
            n177 = property class="Bool"(reference=w392, error in=w393, "Colors [4]"=w388) -> (error out=w390:errorcluster)  [unwired: 1 out]
            n178 = property class="Bool"(reference=w389, error in=w390, "Colors [4]"=w388) -> (error out=w391:errorcluster)  [unwired: 1 out]
          }
        }
        n179 = Format Into String(format string=w325, w352) -> (resulting string=w351:string)  [unwired: 2 in, 1 out]
        n180 = call "Execute query.vi"("error in (no error)"=w355, "String"=w351, "connection reference"=w354) -> ("error out"=w332:errorcluster, "Table"=w313:string[][], "connection reference 2"=w353:T1)  [unwired: 3 in, 3 out]
        n181 = Index Array(array=w313, index (col) #1=0 ("disabled index (col)")) -> (element #1=w315:string[], element #2=w314:string[])  [unwired: 3 in]
        n182 = for {
          tunnel: w315 -> [w363] mode=indexing
          tunnel: w314 -> [w364] mode=indexing
          tunnel: [w362] -> w312 mode=indexing
          n183 = Empty String/Path?(string/path=w363) -> (empty?=w366:bool)
          n184 = Empty String/Path?(string/path=w364) -> (empty?=w367:bool)
          n185 = Or(x=w366, y=w367) -> (x .or. y?=w365:bool)
          n186 = case shown="False" w365 {
            tunnel: [w370 0.0] -> w362
            tunnel: w363 -> [w369 _]
            tunnel: w364 -> [w368 _]
            frame False {
              n187 = call "String to timestamp new.vi"("String Timestamp"=w369) -> ("Timestamp"=w372:timestamp)  [unwired: 10 in]
              n188 = call "String to timestamp new.vi"("String Timestamp"=w368) -> ("Timestamp"=w371:timestamp)  [unwired: 10 in]
              n189 = Max & Min(x=w372, y=w371) -> (max(x,y)=w376:timestamp, min(x,y)=w375:timestamp)
              n190 = To Double Precision Float(number=w376) -> (double precision float=w374:dbl)
              n191 = To Double Precision Float(number=w375) -> (double precision float=w373:dbl)
              n192 = Subtract(x=w374, y=w373) -> (x-y=w370:dbl)
            }
            frame True {
            }
          }
        }
        n193 = Add Array Elements(numeric array=w312) -> (sum=→"Q Duration Min" →"Duration Q":dbl)
        n194 = Merge Errors(w332, w331) -> (w330:errorcluster)
      }
      frame "5" {
        w423 = 0 ("index (row)")
        w426 = 0 ("index (row)")
        (unwired) "Select IS_ACTIVE  From STATION_1_LOG_HISTORY\nWhere LOG_ID='%s' \n\n"
        (unwired) "Select MAX(LOG_ID)  From STATION_1_LOG_HISTORY \n Where PLAN_DATE='%s' And BREAKDOWN_STK_HOLD_ID='5'\n\n"
        (unwired) "Select  BREAKDOWN_IN_TIME,BREAKDOWN_OUT_TIME,DATEDIFF (MINUTE,BREAKDOWN_IN_TIME,BREAKDOWN_OUT_TIME)\nFrom STATION_1_LOG_HISTORY\nWhere PLAN_DATE ='%s'  And BREAKDOWN_STK_HOLD_ID='5'\n\n"  # Select  BREAKDOWN_IN_TIME,BREAKDOWN_OUT_TIME,DATEDIFF (MINUTE,BREAKDOWN_IN_TIME,BREAKDOWN_OUT_TIME) From STATION_1_LOG_HISTORY Where PLAN_DATE ='%s'  And BREAKDOWN_STK_HOLD_ID='5'
        w439 = 0 ("index (row)")
        (unwired) "Select COUNT(LOG_ID)  From STATION_1_LOG_HISTORY \n Where PLAN_DATE='%s' And BREAKDOWN_STK_HOLD_ID='5'"  # Select COUNT(LOG_ID)  From STATION_1_LOG_HISTORY   Where PLAN_DATE='%s' And BREAKDOWN_STK_HOLD_ID='5'
        n195 = Concatenate Strings("Select IS_ACTIVE  From \n\n", w402, " Where LOG_ID='%s' \n\n") -> (w399:string)
        n196 = Concatenate Strings("Select MAX(LOG_ID)  From \n", w402, " Where PLAN_DATE='%s' And BREAKDOWN_STK_HOLD_ID='5'\n\n") -> (w407:string)
        n197 = global read "Current date.vi" "Current Date"() -> (w431:string)
        n198 = Concatenate Strings("Select COUNT(LOG_ID)  From \n", w402, " Where PLAN_DATE='%s' And BREAKDOWN_STK_HOLD_ID='5'\n\n") -> (w400:string)
        n199 = Concatenate Strings("Select  BREAKDOWN_IN_TIME,BREAKDOWN_OUT_TIME,DATEDIFF (MINUTE,BREAKDOWN_IN_TIME,BREAKDOWN_OUT_TIME)\nFROM " ("SQL query"), w402, " Where PLAN_DATE='%s' And BREAKDOWN_STK_HOLD_ID='5'\n\n") -> (w401:string)
        n200 = Format Into String(format string=w407, w431) -> (resulting string=w430:string)  [unwired: 2 in, 1 out]
        n201 = call "Execute query.vi"("error in (no error)"=w421, "String"=w430, "connection reference"=w420) -> ("error out"=w429:errorcluster, "Table"=w425:string[][], "connection reference 2"=w428:T1)  [unwired: 3 in, 3 out]
        n202 = global read "Current date.vi" "Current Date"() -> (w434:string)
        n203 = Index Array(array=w425, index (row)=w426, index (col)=w426) -> (element=w424:string)
        n204 = Format Into String(format string=w399, w424) -> (resulting string=w427:string)  [unwired: 2 in, 1 out]
        n205 = call "Execute query.vi"("error in (no error)"=w429, "String"=w427, "connection reference"=w428) -> ("error out"=w408:errorcluster, "Table"=w422:string[][], "connection reference 2"=w419:T1)  [unwired: 3 in, 3 out]
        n206 = Format Into String(format string=w400, w434) -> (resulting string=w441:string)  [unwired: 2 in, 1 out]
        n207 = Index Array(array=w422, index (row)=w423, index (col)=w423) -> (element=w418:string)
        n208 = call "Execute query.vi"("error in (no error)"=w408, "String"=w441, "connection reference"=w419) -> ("error out"=w437:errorcluster, "Table"=w440:string[][], "connection reference 2"=w436:T1)  [unwired: 3 in, 3 out]
        n209 = control-ref of="P Ack"() -> (w417:refnum<vi>)
        n210 = control-ref of="SS"() -> (w416:refnum<vi>)
        n211 = Index Array(array=w440, index (row)=w439, index (col)=w439) -> (element=w438:string)
        n212 = Decimal String To Number(string=w438) -> (number=→"P Counter" →"COUNT P":i32)  [unwired: 2 in, 1 out]
        n213 = case shown="\"3\", Default" w418 {
          tunnel: [w460 w467 w472] -> w413
          tunnel: w408 -> [w462 w464 w475]
          tunnel: w417 -> [_ w466 w474]
          tunnel: w416 -> [w461 w465 w471]
          frame "1" {
            n214 = property class="Bool"(reference=w461, error in=w462, "Colors [4]"=cluster{u32, u32}[] [{52224, 52224}]) -> (error out=w460:errorcluster)  [unwired: 1 out]
          }
          frame "3", Default {
            w468 = cluster{u32, u32}[] [{12369084, 12369084}] ("Colors [4]")
            n215 = property class="Bool"(reference=w465, error in=w464, "Colors [4]"=w468) -> (error out=w469:errorcluster)  [unwired: 1 out]
            n216 = property class="Bool"(reference=w466, error in=w469, "Colors [4]"=w468) -> (error out=w467:errorcluster)  [unwired: 1 out]
          }
          frame "2" {
            w470 = cluster{u32, u32}[] [{52224, 52224}] ("Colors [4]")
            n217 = property class="Bool"(reference=w474, error in=w475, "Colors [4]"=w470) -> (error out=w473:errorcluster)  [unwired: 1 out]
            n218 = property class="Bool"(reference=w471, error in=w473, "Colors [4]"=w470) -> (error out=w472:errorcluster)  [unwired: 1 out]
          }
        }
        n219 = Format Into String(format string=w401, w434) -> (resulting string=w433:string)  [unwired: 2 in, 1 out]
        n220 = call "Execute query.vi"("error in (no error)"=w437, "String"=w433, "connection reference"=w436) -> ("error out"=w415:errorcluster, "Table"=w395:string[][], "connection reference 2"=w435:T1)  [unwired: 3 in, 3 out]
        n221 = Index Array(array=w395, index (col) #1=0 ("disabled index (col)")) -> (element #1=w397:string[], element #2=w396:string[])  [unwired: 3 in]
        n222 = for {
          tunnel: w397 -> [w445] mode=indexing
          tunnel: w396 -> [w446] mode=indexing
          tunnel: [w444] -> w394 mode=indexing
          n223 = Empty String/Path?(string/path=w445) -> (empty?=w448:bool)
          n224 = Empty String/Path?(string/path=w446) -> (empty?=w449:bool)
          n225 = Or(x=w448, y=w449) -> (x .or. y?=w447:bool)
          n226 = case shown="False" w447 {
            tunnel: [w452 0.0] -> w444
            tunnel: w445 -> [w451 _]
            tunnel: w446 -> [w450 _]
            frame False {
              n227 = call "String to timestamp new.vi"("String Timestamp"=w451) -> ("Timestamp"=w454:timestamp)  [unwired: 10 in]
              n228 = call "String to timestamp new.vi"("String Timestamp"=w450) -> ("Timestamp"=w453:timestamp)  [unwired: 10 in]
              n229 = Max & Min(x=w454, y=w453) -> (max(x,y)=w458:timestamp, min(x,y)=w457:timestamp)
              n230 = To Double Precision Float(number=w458) -> (double precision float=w456:dbl)
              n231 = To Double Precision Float(number=w457) -> (double precision float=w455:dbl)
              n232 = Subtract(x=w456, y=w455) -> (x-y=w452:dbl)
            }
            frame True {
            }
          }
        }
        n233 = Add Array Elements(numeric array=w394) -> (sum=→"P Duration Min" →"Duration P":dbl)
        n234 = Merge Errors(w415, w413) -> (w414:errorcluster)
      }
    }
    n235 = Wait (ms)(milliseconds to wait=u32 100) -> ()  [unwired: 1 out]
  }
  n236 = property class="App"(error in=w29) -> (error out=w30:errorcluster, "App.Kind"=w31:T2)  [unwired: 1 in, 1 out]
  n237 = call <vilib>:"DB Tools Close Connection.vi"("connection reference"=w2) -> ("error out"=w1:errorcluster)  [unwired: 6 in]
  n238 = Unbundle By Name(w1) -> ()  [unwired: 1 out]
  n239 = case shown="\"Run Time System\"" w31 {
    tunnel: w30 -> [w477 w482]
    tunnel: [w476 w481] -> w7
    frame Default {
      n240 = disable-structure shown="Enabled" {
        disable-tunnel: w477 -> [w479 w480]
        disable-tunnel: [w478 w480] -> w476
        frame Disabled {
          n241 = invoke class="VI" method="FP.Close"(error in=w479) -> (error out=w478:errorcluster)  [unwired: 2 in, 2 out]
        }
        frame Enabled {
        }
      }
    }
    frame "Run Time System" {
      n242 = invoke class="VI" method="FP.Close"(error in=w482) -> (error out=w481:errorcluster)  [unwired: 2 in, 2 out]
    }
  }
  "error out" <- w7
